vi "X10translator.vi"(0 "Unit No.":i32=1 min=1 max=16, 1 "House Code":i32(ring)=1 items=["-----", "A", "B", "C", "D", "E", "F", "G", "H", "I", "J", "K", "L", "M", "N", "O", "P"], 2 "Function Codes (ON)":u8(ring)=2 items=["All lights OFF", "All lights ON", "ON", "OFF", "Dim", "Bright", "All lights OFF", "Extended Code", "Hail Request", "Hail Acknowledge", "Pre-set Dim (1)", "Pre-set Dim (2)", "Extended data transfer", "Status ON", "Status OFF", "Status Request"], 5 "Transmission type (address)":enum8{"Address", "Function"}(ring), 6 "Number of \"Dims\"(0)":u8 max=22, 7 "Transmission length (standard)":enum8{"Standard", "Extended"}(ring)) -> (3 "checksum":string, 4 "Send string":string)   [LabVIEW 2010]
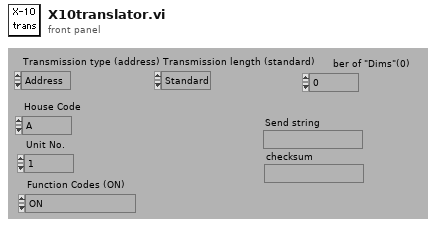
[diagram p1: front panel]
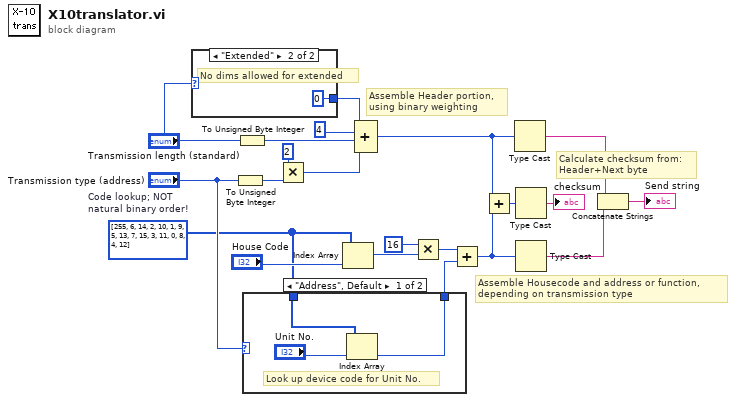
[diagram p0: block diagram]
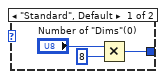
[diagram p2: hidden frame]
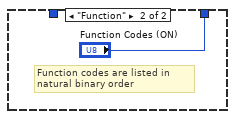
[diagram p3: hidden frame]
diagram:
  w14 = u8[] [255, 6, 14, 2, 10, 1, 9, 5, 13, 7, 15, 3, 11, 0, 8, 4, 12]  # Code lookup; NOT natural binary order!
  # "Calculate checksum from:\nHeader+Next byte"
  # "Assemble Housecode and address or function,\ndepending on transmission type"
  # "Assemble Header portion,\nusing binary weighting"
  n1 = case shown="\"Extended\"" "Transmission length (standard)" {
    tunnel: [w23 u8 0] -> w20
    frame "Standard", Default {
      n2 = Multiply(x="Number of \"Dims\"(0)", y=u8 8) -> (x*y=w23:u8)
    }
    frame "Extended" {
      # "No dims allowed for extended"
    }
  }
  n3 = To Unsigned Byte Integer(number="Transmission type (address)") -> (unsigned 8bit integer=w1:u8)
  n4 = To Unsigned Byte Integer(number="Transmission length (standard)") -> (unsigned 8bit integer=w2:u8)
  n5 = case shown="\"Address\", Default" "Transmission type (address)" {
    tunnel: [w26 "Function Codes (ON)"] -> w10
    tunnel: w14 -> [w27 _]
    frame "Address", Default {
      # "Look up device code for Unit No."
      n6 = Index Array(array=w27, index="Unit No.") -> (element=w26:u8)
    }
    frame "Function" {
      # "Function codes are listed in natural binary order"
    }
  }
  n7 = Multiply(x=u8 2, y=w1) -> (x*y=w17:u8)
  n8 = Index Array(array=w14, index="House Code") -> (element=w13:u8)
  n9 = Compound Arithmetic op=ADD(w20, u8 4 ("y"), w2, w17) -> (w3:u8)
  n10 = Multiply(x=u8 16, y=w13) -> (x*y=w11:u8)
  n11 = Add(x=w11, y=w10) -> (x+y=w8:u8)
  n12 = Add(x=w3, y=w8) -> (x+y=w5:u8)
  n13 = Type Cast(x=w3) -> (*(type *) &x=w9:string)  [unwired: 1 out]
  n14 = Type Cast(x=w5) -> (*(type *) &x=→"checksum":string)  [unwired: 1 out]
  n15 = Type Cast(x=w8) -> (*(type *) &x=w7:string)  [unwired: 1 out]
  n16 = Concatenate Strings(w9, w7) -> (→"Send string":string)
